vi "RunFPGA.vi"(8 "error in":errorcluster, 11 "FPGASession in":refnum<class "FPGASession.lvclass">) -> (0 "error out":errorcluster, 3 "FPGASession out":refnum<class "FPGASession.lvclass">)   [LabVIEW 2013, in "FPGASession.lvclass"]
uses:
  FPGASession.lvclass
  FPGASession.lvclass/FPGASession.ctl
  <vilib>/rvi/interface/nirviMethod/nirviMethod.xnode
  RT/FPGASession/FPGARef.ctl
  FPGA Bitfiles/HWSWTriggerBox_FPGATarget2_TriggerBox_1zhzIx5zPP8.lvbitx
  FPGAMain.vi
  <vilib>/FPGAPlugInAG/sbRIO-9636/niLvFpga_Abort_sbRIO-9636.vi
  <vilib>/FPGAPlugInAG/sbRIO-9636/niLvFpga_Reset_sbRIO-9636.vi
  <vilib>/FPGAPlugInAG/sbRIO-9636/niLvFpga_Run_sbRIO-9636.vi
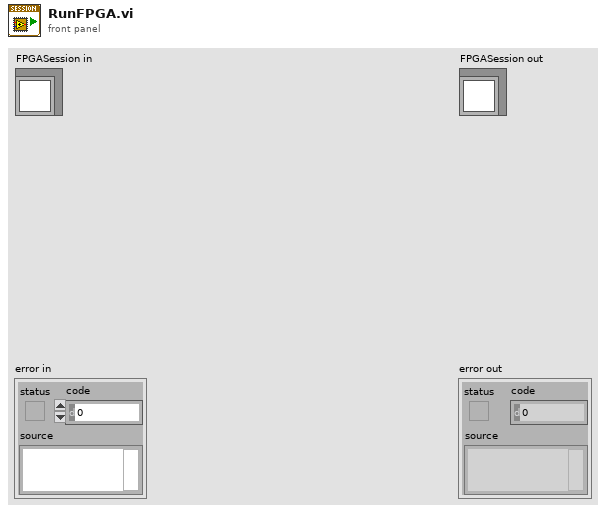
[diagram p1: front panel]
types:
  T1 = typedef "FPGASession.lvclass/FPGARef.ctl" = refnum<k20>
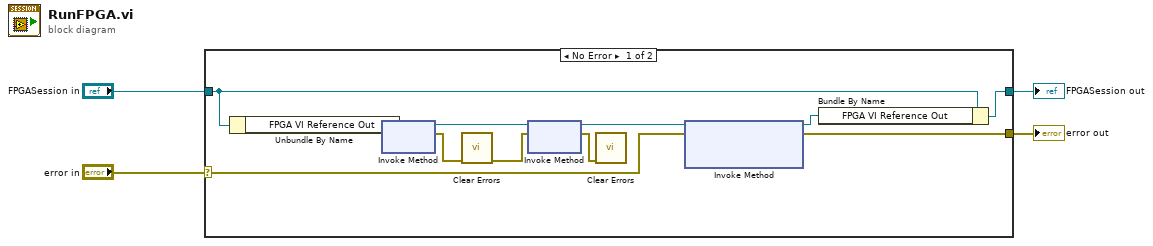
[diagram p0: block diagram]
diagram:
  n1 = case shown="No Error" "error in" {
    selector: "error in" -> [w13 w17]
    tunnel: [w14 w17] -> w4
    tunnel: [w11 w16] -> w2
    tunnel: "FPGASession in" -> [w9 w16]
    frame No Error {
      n2 = Unbundle By Name(w9) -> ("FPGA VI Reference Out"=w12:T1)
      n3 = xnode "Invoke Method"("FPGA VI Reference In"=w12) -> ("FPGA VI Reference Out"=w8:T1, "error out"=w15:errorcluster)  [unwired: 1 in]
      n4 = call <vilib>:"Clear Errors.vi"("error in (no error)"=w15) -> ("error out"=w6:errorcluster)  [unwired: 6 in]
      n5 = xnode "Invoke Method"("FPGA VI Reference In"=w8, "error in"=w6) -> ("FPGA VI Reference Out"=w7:T1, "error out"=w5:errorcluster)
      n6 = call <vilib>:"Clear Errors.vi"("error in (no error)"=w5) -> ()  [unwired: 6 in, 1 out]
      n7 = xnode "Invoke Method"("FPGA VI Reference In"=w7, "error in"=w13) -> ("FPGA VI Reference Out"=w10:T1, "error out"=w14:errorcluster)  [unwired: 1 in]
      n8 = Bundle By Name(cluster=w9, "FPGA VI Reference Out"=w10) -> (w11:refnum<class "FPGASession.lvclass">)
    }
    frame Error {
    }
  }
  "error out" <- w4
  "FPGASession out" <- w2
